vi "Get Active Buffer.vi"(8 "error in (no error)":errorcluster, 11 "Transfer Group in":refnum<class "Transfer Group.lvclass">) -> (0 "error out":errorcluster, 2 "Buffer":refnum<class "Buffer.lvclass">, 3 "Transfer Group out":refnum<class "Transfer Group.lvclass">)   [LabVIEW 2017, in "DSF Core.lvlib" / "Transfer Group.lvclass"]
uses:
  Transfer Group.lvclass
  Buffer/Buffer.lvclass
  Transfer Group.lvclass/Transfer Group.ctl
  Buffers/Buffers.lvclass
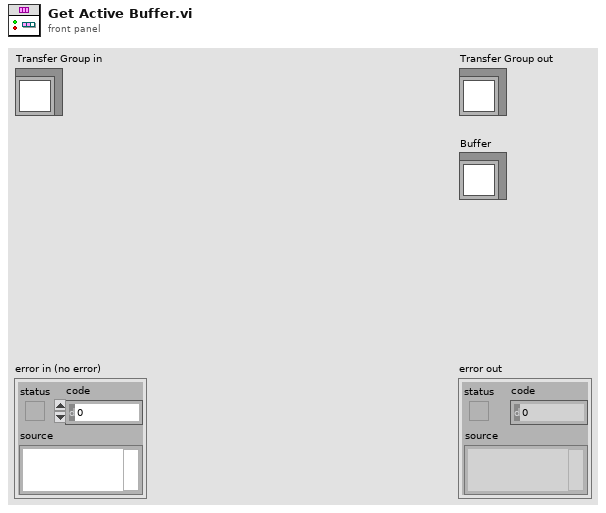
[diagram p1: front panel]
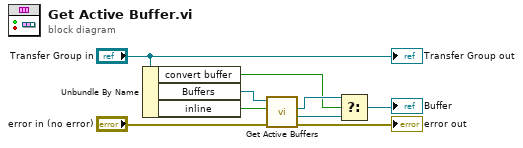
[diagram p0: block diagram]
diagram:
  n1 = Unbundle By Name("Transfer Group in") -> ("convert buffer"=w1:bool, "Buffers"=w9:refnum<class "Buffers.lvclass">, "inline"=w6:bool)
  n2 = call "Get Active Buffers.vi"("error in (no error)"="error in (no error)", "inline?"=w6, "Buffers in"=w9) -> ("error out"=→"error out":errorcluster, "engine Buffer"=w2:refnum<class "Buffer.lvclass">, "string Buffer"=w3:refnum<class "Buffer.lvclass">)  [unwired: 5 in, 1 out]
  n3 = Select(t=w3, s=w1, f=w2) -> (s? t:f=→"Buffer":refnum<class "Buffer.lvclass">)
  "Transfer Group out" <- "Transfer Group in"
